vi "UpdateSystemInfoToMap.vi"(8 "error in (no error)":errorcluster, 11 "map in":T2) -> (0 "error out":errorcluster, 1 "hostname":string, 2 "system info":T1, 3 "map Out":T2, 5 "firmware rev":string)   [LabVIEW 2017, in "SystemInfoProcess.lvlib"]
uses:
  <vilib>/addons/SystemInfoProcess/SystemInfoProcess.lvlib
  <vilib>/addons/PointValueMap/controls/PointMap.ctl
  <vilib>/addons/SystemInfoProcess/controls/ImageMetadata.ctl
  <vilib>/addons/PointValueMap/subVIs/Point_Write_string.vi
  <vilib>/addons/PointValueMap/subVIs/Point_Write_variant.vi
  <resource>/objmgr/nisysapi.rc
  <vilib>/addons/PointValueMap/PointValueMap.lvlib
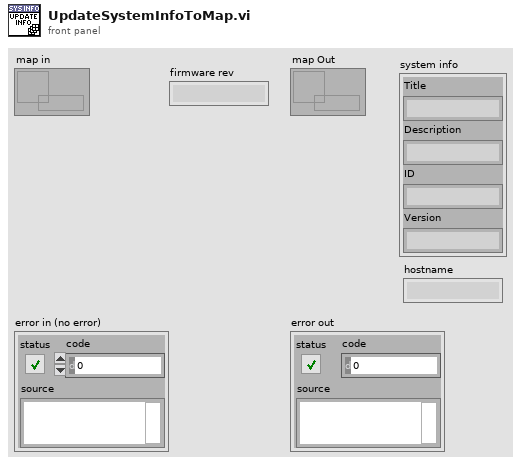
[diagram p1: front panel]
types:
  T1 = typedef "SystemInfoProcess.lvlib/ImageMetadata.ctl" = cluster{"Title":string, "Description":string, "ID":string, "Version":string}
  T2 = typedef "PointValueMap.lvlib/PointMap.ctl" = refnum<data-value>
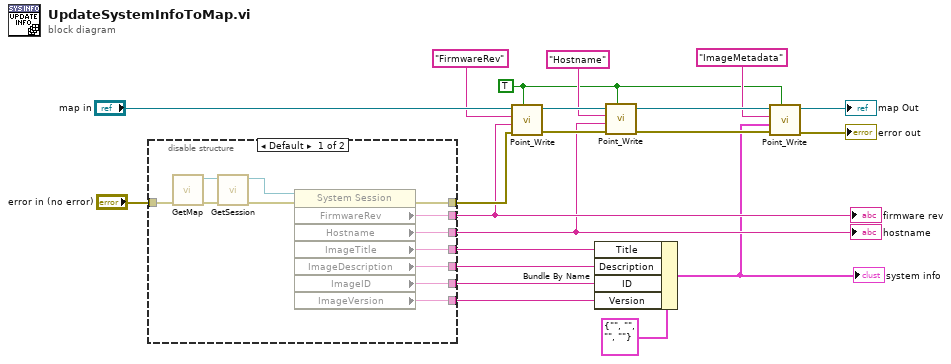
[diagram p0: block diagram]
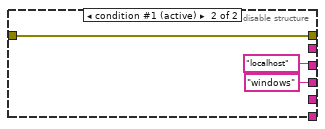
[diagram p2: hidden frame]
diagram:
  w9 = TRUE ("Auto Create?")
  n1 = disable-structure shown="Default" {
    disable-tunnel: "error in (no error)" -> [w24 w36]
    disable-tunnel: [w33 w36] -> w19
    disable-tunnel: [w32 _] -> w18
    disable-tunnel: [w31 "localhost" ("hostname")] -> w15
    disable-tunnel: [w30 "windows" ("ImageTitle")] -> w7
    disable-tunnel: [w29 _] -> w6
    disable-tunnel: [w28 _] -> w5
    disable-tunnel: [w27 _] -> w4
    frame condition #0 {
      n2 = call <vilib>:"GetMap.vi"("error in (no error)"=w24) -> ("error out"=w23:errorcluster, "SystemInfoMap"=w22:T2)  [unwired: 9 in]
      n3 = call <vilib>:"GetSession.vi"("error in (no error)"=w23, "map"=w22) -> ("error out"=w26:errorcluster, "session"=w25:refnum<k21>)  [unwired: 8 in]
      n4 = property class="System Session"(reference=w25, error in=w26) -> (error out=w33:errorcluster, "FirmwareRev"=w32:string, "Hostname"=w31:string, "ImageTitle"=w30:string, "ImageDescription"=w29:string, "ImageID"=w28:string, "ImageVersion"=w27:string)  [unwired: 1 out]
    }
    frame condition #1 (active) {
    }
  }
  "hostname" <- w15
  "firmware rev" <- w18
  n5 = call-poly <vilib>:"Point_Write.vi"("Auto Create?"=w9, "Error In"=w19, "Value"=w18, "Tag"="FirmwareRev", "Map"="map in") -> ("Error Out"=w17:errorcluster, "Map Out"=w16:T2)  [unwired: 5 in]
  n6 = Bundle By Name(cluster=T1 {"Title"="", "Description"="", "ID"="", "Version"=""} ("ImageMetadata"), "Title"=w7, "Description"=w6, "ID"=w5, "Version"=w4) -> (w3:T1)
  "system info" <- w3
  n7 = call-poly <vilib>:"Point_Write.vi"("Auto Create?"=w9, "Error In"=w17, "Value"=w15, "Tag"="Hostname", "Map"=w16) -> ("Error Out"=w12:errorcluster, "Map Out"=w11:T2)  [unwired: 5 in]
  n8 = call-poly <vilib>:"Point_Write.vi"("Auto Create?"=w9, "Error In"=w12, "Value"=w3, "Tag"="ImageMetadata", "Map"=w11) -> ("Error Out"=→"error out":errorcluster, "Map Out"=→"map Out":T2)  [unwired: 5 in]
